vi "TB-Brickwall Noise.vi"(7 "InvFilt Params":T1={"Min Frequency (Hz)"=0.0, "Max Frequency (Hz)"=0.0, "Length (points)"=301, "Sampling rate (Hz)"=0.0, "Delay (ms)"=301.0, "Linear phase"=FALSE}, 11 "error in (no error)":errorcluster) -> (4 "InvFilter Noise":dbl[](array[numeric]), 15 "error out":errorcluster)   [LabVIEW 2020]
uses:
  epl-cal-vi-lib/Inverse Filter VIs/InvFilt-Params.ctl
  epl-vi-lib/Utility VIs/Math VIs/FFT x(t) to dB,Degrees (1D).vi
  <vilib>/Analysis/NI_AALBase.lvlib
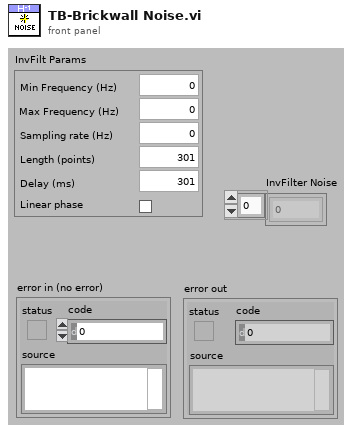
[diagram p1: front panel]
types:
  T1 = typedef "InvFilt-Params.ctl" = cluster{"Min Frequency (Hz)":dbl, "Max Frequency (Hz)":dbl, "Length (points)":i32, "Sampling rate (Hz)":dbl, "Delay (ms)":dbl, "Linear phase":bool}
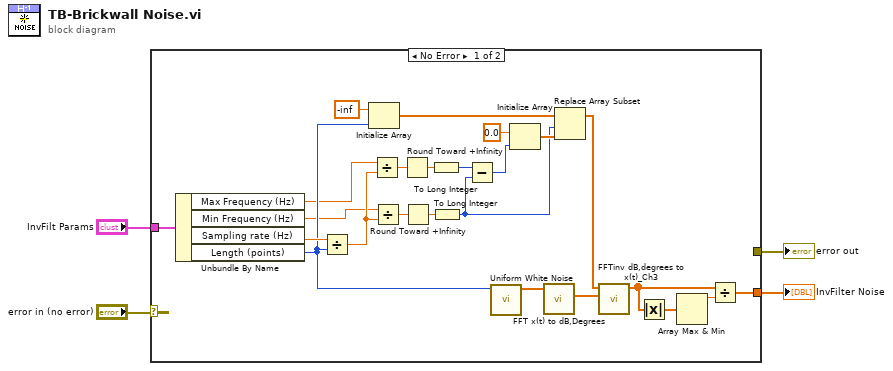
[diagram p0: block diagram]
diagram:
  n1 = case shown="No Error" "error in (no error)" {
    selector: "error in (no error)" -> [_ w29]
    tunnel: [_ w29] -> w3
    tunnel: "InvFilt Params" -> [w28 _]
    tunnel: [w22 _] -> w1
    frame No Error {
      n2 = Unbundle By Name(w28) -> ("Max Frequency (Hz)"=w9:dbl, "Min Frequency (Hz)"=w8:dbl, "Sampling rate (Hz)"=w11:dbl, "Length (points)"=w10:i32)
      n3 = Divide(x=w11, y=w10) -> (x/y=w18:dbl)
      n4 = Initialize Array(-inf ("element"), w10) -> (w6:dbl[])
      n5 = Divide(x=w9, y=w18) -> (x/y=w12:dbl)
      n6 = Divide(x=w8, y=w18) -> (x/y=w14:dbl)
      n7 = Round Toward +Infinity(x=w12) -> (ceil(x): smallest int >= x=w13:dbl)
      n8 = Round Toward +Infinity(x=w14) -> (ceil(x): smallest int >= x=w15:dbl)
      n9 = To Long Integer(number=w13) -> (32bit integer=w7:i32)
      n10 = To Long Integer(number=w15) -> (32bit integer=w16:i32)
      n11 = Subtract(x=w7, y=w16) -> (x-y=w17:i32)
      n12 = call <vilib>:"Uniform White Noise.vi"("samples"=w10) -> ("uniform white noise"=w23:dbl[])  [unwired: 9 in, 1 out]
      n13 = Initialize Array(0.0 ("element"), w17) -> (w20:dbl[])
      n14 = call-poly "FFT x(t) to dB,Degrees.vi"("X"=w23) -> ("+Freq Phase of FFT (degrees)"=w27:dbl[])  [unwired: 8 in, 2 out]
      n15 = Replace Array Subset(array=w6, new element=w20, index=w16) -> (w5:dbl[])
      n16 = call "FFTinv dB,degrees to x(t)_Ch3.vi"("+Freq Phase of FFT (degrees)"=w27, "+Freq. Mag of FFT (rms dB)"=w5) -> ("X(t)"=w24:dbl[])  [unwired: 8 in, 1 out]
      n17 = Absolute Value(x=w24) -> (abs(x)=w26:dbl[])
      n18 = Array Max & Min(array=w26) -> (max value=w25:dbl)  [unwired: 3 out]
      n19 = Divide(x=w24, y=w25) -> (x/y=w22:dbl[])
    }
    frame Error {
    }
  }
  "error out" <- w3
  "InvFilter Noise" <- w1
